vi "CheckGameBoardGetNeighbours.vi"(8 "error in (no error)":errorcluster, 10 "Position in":cluster{"row":i32, "column":i32}, 11 "Board size(s)":i32[](array[numeric])) -> (0 "error out":errorcluster, 3 "Positions out":cluster{"row":i32, "column":i32}[](array[cluster]))   [LabVIEW 2020]
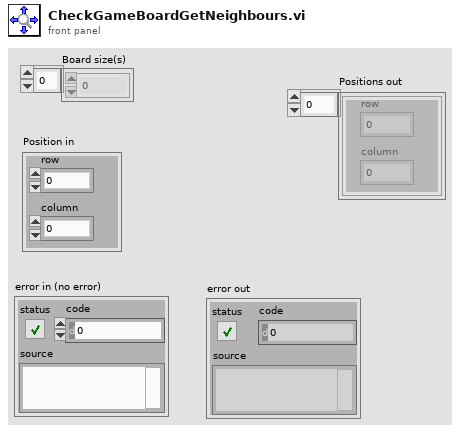
[diagram p1: front panel]
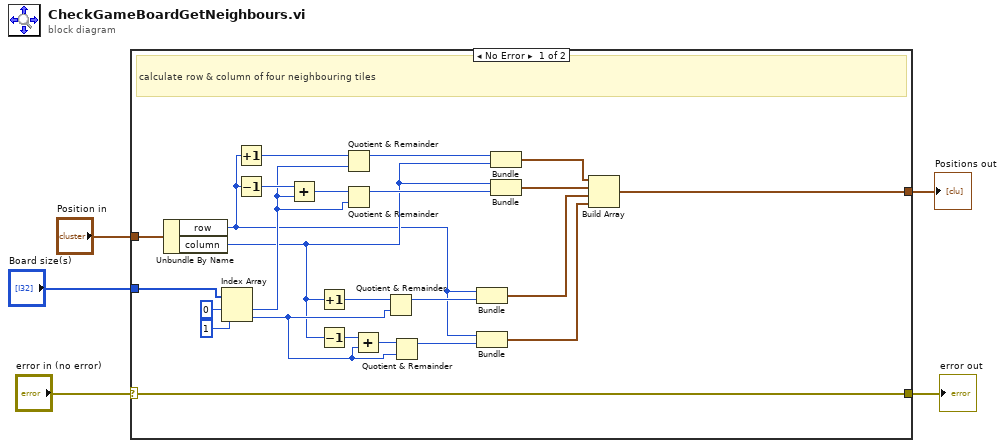
[diagram p0: block diagram]
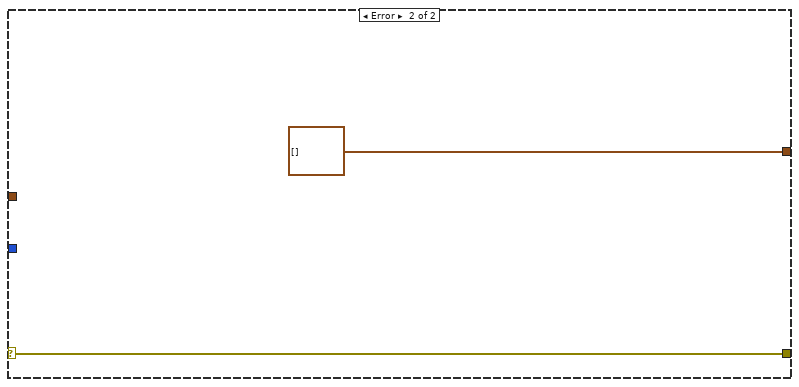
[diagram p2: hidden frame]
diagram:
  n1 = case shown="No Error" "error in (no error)" {
    selector: "error in (no error)" -> [w28 w31]
    tunnel: "Position in" -> [w29 _]
    tunnel: [w28 w31] -> w3
    tunnel: [w12 cluster{i32, i32}[] []] -> w2
    tunnel: "Board size(s)" -> [w6 _]
    frame No Error {
      # "calculate row & column of four neighbouring tiles"
      n2 = Unbundle By Name(w29) -> ("row"=w7:i32, "column"=w10:i32)
      n3 = Index Array(array=w6, index #1=0 ("index"), index #2=1 ("index")) -> (element #1=w23:i32, element #2=w18:i32)
      n4 = Increment(x=w7) -> (x+1=w20:i32)
      n5 = Decrement(x=w7) -> (x-1=w25:i32)
      n6 = Add(x=w25, y=w23) -> (x+y=w24:i32)
      n7 = Increment(x=w10) -> (x+1=w19:i32)
      n8 = Decrement(x=w10) -> (x-1=w22:i32)
      n9 = Quotient & Remainder(x=w20, y=w23) -> (x-y*floor(x/y)=w17:i32)  [unwired: 1 out]
      n10 = Quotient & Remainder(x=w24, y=w23) -> (x-y*floor(x/y)=w11:i32)  [unwired: 1 out]
      n11 = Add(x=w22, y=w18) -> (x+y=w21:i32)
      n12 = Quotient & Remainder(x=w19, y=w18) -> (x-y*floor(x/y)=w9:i32)  [unwired: 1 out]
      n13 = Quotient & Remainder(x=w21, y=w18) -> (x-y*floor(x/y)=w8:i32)  [unwired: 1 out]
      n14 = Bundle("row"=w7, w9) -> (w14:cluster{"row":i32, i32})  [unwired: 1 in]
      n15 = Bundle("row"=w7, w8) -> (w13:cluster{"row":i32, i32})  [unwired: 1 in]
      n16 = Bundle(w17, "column"=w10) -> (w16:cluster{i32, "column":i32})  [unwired: 1 in]
      n17 = Bundle("column"=w10, w11) -> (w15:cluster{"column":i32, i32})  [unwired: 1 in]
      n18 = Build Array(w16, w15, w14, w13) -> (w12:cluster{"row":i32, "column":i32}[])
    }
    frame Error {
    }
  }
  "error out" <- w3
  "Positions out" <- w2
